vi "get_working_distance.vi"(8 "error in (no error)":errorcluster, 11 "GenericObjective in":refnum<class "GenericObjective.lvclass">) -> (0 "error out":errorcluster, 2 "working distance":dbl[unit], 3 "GenericObjective out":refnum<class "GenericObjective.lvclass">)   [LabVIEW 2010, in "GenericObjective.lvclass"]
uses:
  GenericObjective.lvclass
  GenericObjective.lvclass/GenericObjective.ctl
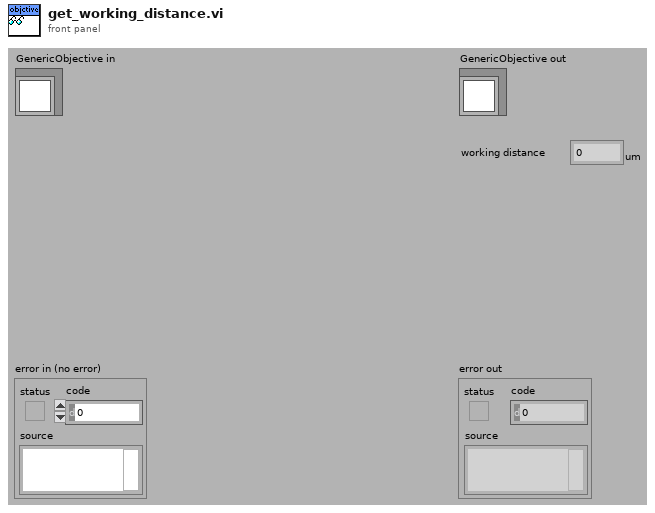
[diagram p1: front panel]
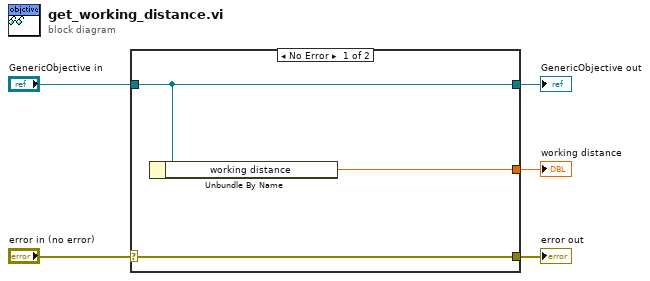
[diagram p0: block diagram]
diagram:
  n1 = case shown="No Error" "error in (no error)" {
    selector: "error in (no error)" -> [w8 w9]
    tunnel: [w8 w9] -> w4
    tunnel: [w7 w10] -> w2
    tunnel: "GenericObjective in" -> [w7 w10]
    tunnel: [w6 _] -> w1
    frame No Error {
      n2 = Unbundle By Name(w7) -> ("working distance"=w6:dbl[unit])
    }
    frame Error {
    }
  }
  "error out" <- w4
  "GenericObjective out" <- w2
  "working distance" <- w1
